vi "exnSpectralBlock spectral measurements PSD DDT.vi"(0 "Signals":dynamicdata(graph), 5 "Restart Averaging":bool, 7 "View":T2, 9 "Spectrum Window":u16, 11 "error in (no error)":errorcluster, 12 "Spectrum Averaging Parameters":T1={"averaging mode"=0, "weighting mode"=1, "number of averages"=10} {"averaging mode" items=["No averaging", "Vector averaging", "RMS averaging", "Peak hold"]; "weighting mode" items=["Linear", "Exponential"]}, 14 "All Spectra":bool) -> (4 "Measurement Output":dynamicdata(graph), 6 "averaging done":bool, 15 "error out":errorcluster)   [LabVIEW 2020]
uses:
  <vilib>/measure/NI_MAPro.lvlib
panel:
  in  "measurement":string="PSD"
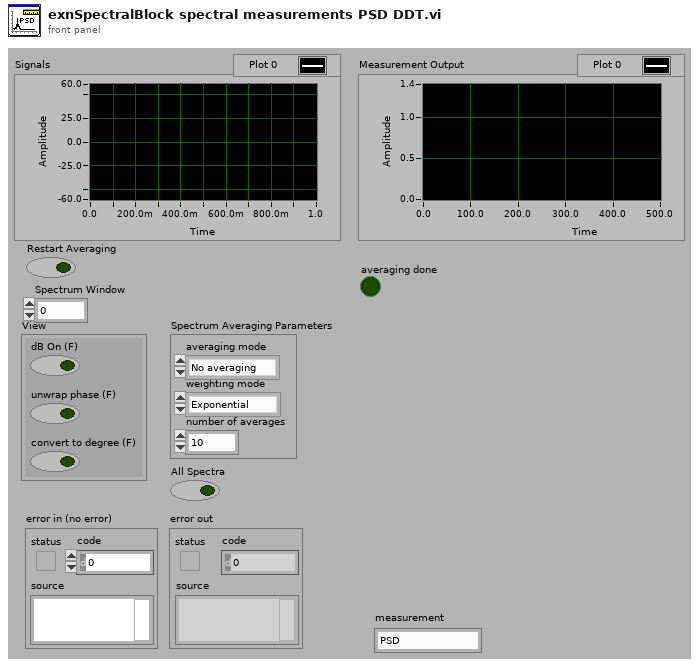
[diagram p1: front panel]
types:
  T1 = cluster{"averaging mode":u16, "weighting mode":u16, "number of averages":u32}
  T2 = cluster{"dB On (F)":bool, "unwrap phase (F)":bool, "convert to degree (F)":bool}
  T3 = enum16{"None ", "Hanning", "Hamming", "Blackman-Harris", "Exact Blackman", "Blackman", "Flat Top", "4 Term B-Harris ", "7 Term B-Harris", "Low Sidelobe"}
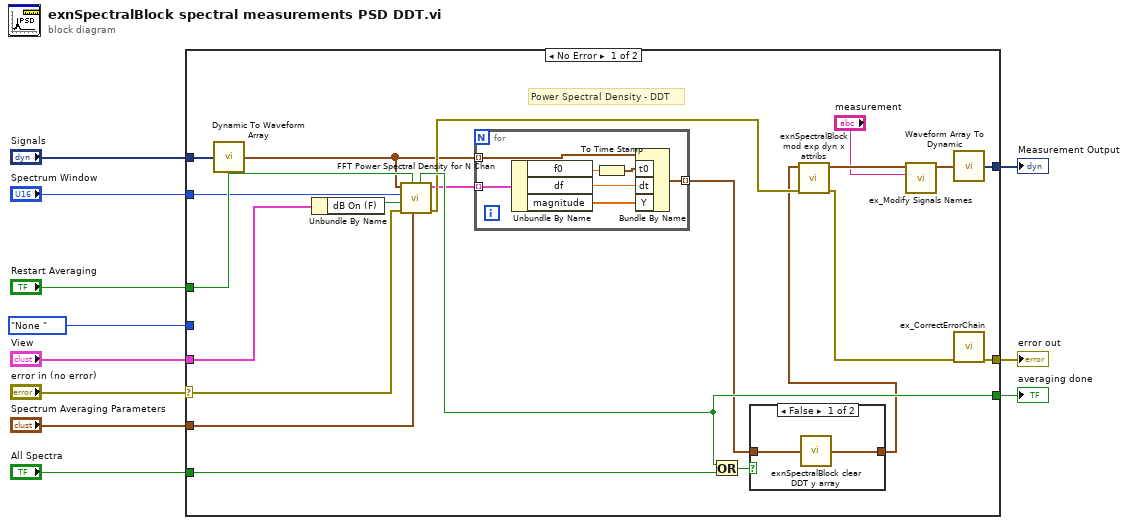
[diagram p0: block diagram]
diagram:
  n1 = case shown="No Error" "error in (no error)" {
    selector: "error in (no error)" -> [w16 w43]
    tunnel: [w32 _] -> w11
    tunnel: [w31 _] -> w10
    tunnel: "All Spectra" -> [w30 _]
    tunnel: "Spectrum Averaging Parameters" -> [w29 _]
    tunnel: "Restart Averaging" -> [w28 _]
    tunnel: T3."None " ("window") -> [_ _]
    tunnel: "Spectrum Window" -> [w17 _]
    tunnel: "View" -> [w27 _]
    tunnel: "Signals" -> [w25 _]
    tunnel: [w24 w43] -> w3
    frame No Error {
      # "Power Spectral Density - DDT"
      n2 = call <vilib>:"Dynamic To Waveform Array.vi"("Input"=w25) -> ("Output"=w18:waveform(dbl)[])  [unwired: 4 in]
      n3 = Unbundle By Name(w27) -> ("dB On (F)"=w14:bool)
      n4 = call <vilib>:"FFT Power Spectral Density for N Chan.vi"("averaging parameters"=w29, "restart averaging (F)"=w28, "error in (no error)"=w16, "dB On (F)"=w14, "window"=w17, "time signals"=w18) -> ("error out"=w26:errorcluster, "power spectral densities"=w13:cluster{"f0":dbl, "df":dbl, "magnitude":dbl[]}[], "averaging done"=w31:bool)  [unwired: 2 in, 1 out]
      n5 = for {
        tunnel: w18 -> [w35] mode=indexing
        tunnel: [w36] -> w20 mode=indexing
        tunnel: w13 -> [w34] mode=indexing
        n6 = Unbundle By Name(w34) -> ("f0"=w39:dbl, "df"=w38:dbl, "magnitude"=w37:dbl[])
        n7 = To Time Stamp(1:w39) -> (0:w33:timestamp)
        n8 = Bundle By Name(cluster=w35, "t0"=w33, "dt"=w38, "Y"=w37) -> (w36:waveform(dbl))
      }
      n9 = Or(x=w31, y=w30) -> (x .or. y?=w21:bool)
      n10 = case shown="False" w21 {
        tunnel: w20 -> [w41 w42]
        tunnel: [w40 w42] -> w19
        frame False {
          n11 = call <vilib>:"exnSpectralBlock clear DDT y array.vi"("Array In"=w41) -> ("Array Out"=w40:waveform(dbl)[])
        }
        frame True {
        }
      }
      n12 = call <vilib>:"exnSpectralBlock mod exp dyn x attribs.vi"("error in (no error)"=w26, "Signals in"=w19) -> ("error out"=w12:errorcluster, "Signals out"=w23:waveform(dbl)[])  [unwired: 8 in]
      n13 = call <vilib>:"ex_Modify Signals Names.vi"("Name Modifier"="measurement", "Array of Waveforms In"=w23) -> ("Array of Waveforms Out"=w22:waveform(dbl)[])  [unwired: 8 in, 1 out]
      n14 = call <vilib>:"Waveform Array To Dynamic.vi"("Input"=w22) -> ("Output"=w32:dynamicdata)  [unwired: 4 in]
      n15 = call <vilib>:"ex_CorrectErrorChain.vi"("error in (no error)"=w12) -> ("error out"=w24:errorcluster)  [unwired: 10 in]
    }
    frame Error {
    }
  }
  "Measurement Output" <- w11
  "averaging done" <- w10
  "error out" <- w3
